vi "Read Field Interpolate.vi"(8 "error in (no error)":errorcluster, 11 "input cluster":T1) -> (0 "error out":errorcluster, 2 "Field (T)":dbl format="%_6f", 3 "output cluster":T1)   [LabVIEW 2012]
uses:
  Magna Power Constants.vi
  <vilib>/gmath/NI_Gmath.lvlib
panel:
  out "Fluke Voltage (V)":dbl format="%.6f"
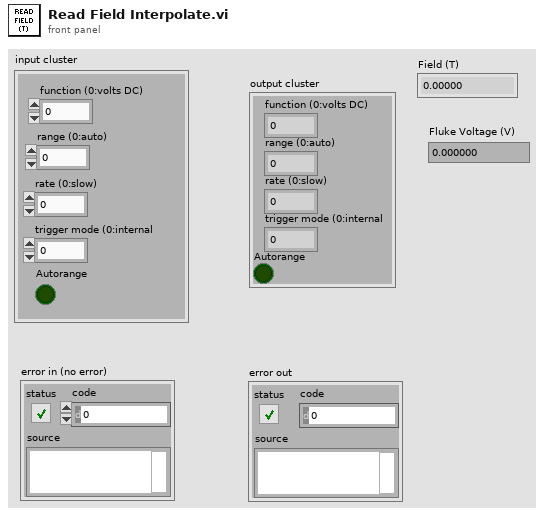
[diagram p1: front panel]
types:
  T1 = cluster{"function (0:volts DC)":i16, "range (0:auto)":i16, "rate (0:slow)":i16, "trigger mode (0:internal":i16, "Autorange":bool}
  T2 = cluster{"Magna Current":dbl[], "Magnetic Field":dbl[], "Fluke Voltage":dbl[]}
  T3 = cluster{"function (0:volts DC)":u16, "range (0:auto)":u16, "rate (0:slow)":u16, "trigger mode (0:internal)":u16, "Autorange":bool}
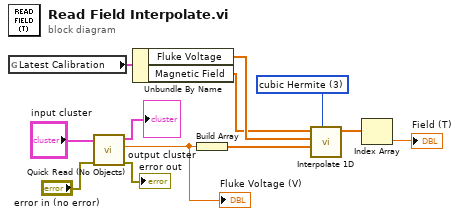
[diagram p0: block diagram]
diagram:
  w1 = 3 items=["nearest", "linear", "spline", "cubic Hermite", "Lagrange"] ("method")
  n1 = global read "Magna Power Constants.vi" "Latest Calibration"() -> (w12:T2)
  n2 = call "Quick Read (No Objects).vi"("error in (no error)"="error in (no error)", "Fluke Multimeter In"="input cluster") -> ("error out"=→"error out":errorcluster, "measurement"=w5:dbl, "Fluke Multimeter Out"=→"output cluster":T3)  [unwired: 6 in, 1 out]
  "Fluke Voltage (V)" <- w5
  n3 = Unbundle By Name(w12) -> ("Fluke Voltage"=w7:dbl[], "Magnetic Field"=w6:dbl[])
  n4 = Build Array(w5) -> (w4:dbl[])
  n5 = call <vilib>:"Interpolate 1D.vi"("method"=w1, "xi"=w4, "X"=w7, "Y"=w6) -> ("yi"=w3:dbl[])  [unwired: 5 in, 2 out]
  n6 = Index Array(array=w3) -> (element=→"Field (T)":dbl)  [unwired: 1 in]
